vi "csm_lumikki_instron_startRamp_poller.vi"   [LabVIEW 2009]
types:
  T1 = cluster{"Device ID":i32, "Device Name":string, "Device Type":i32}[]
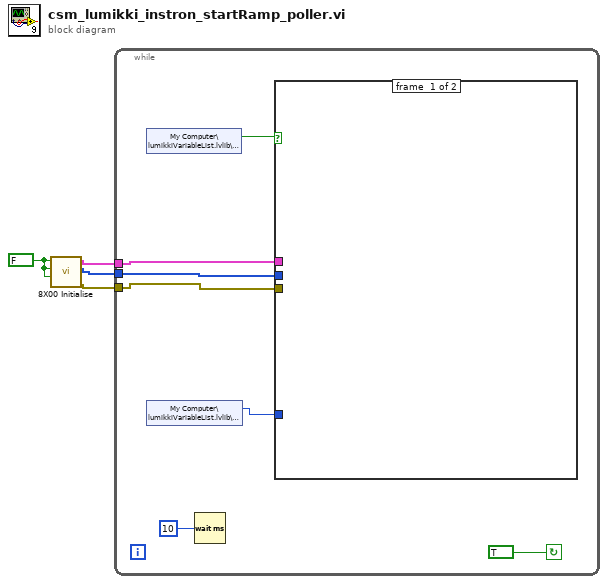
[diagram p0: block diagram]
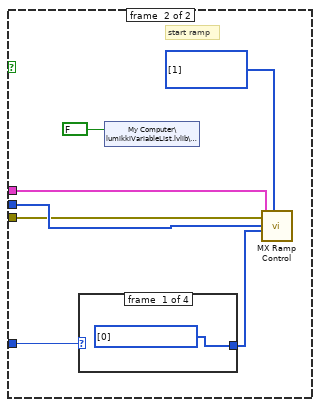
[diagram p2: hidden frame]
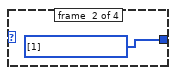
[diagram p3: hidden frame]
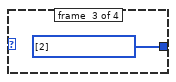
[diagram p4: hidden frame]
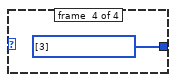
[diagram p5: hidden frame]
diagram:
  w4 = FALSE ("Create Console? (T)")
  n1 = call "8X00 Initialise.vi"("Reset?"=w4, "Create DVM? (T)"=w4, "Create Console? (T)"=w4) -> ("error out"=w1:errorcluster, "Axis Selector"=w2:i32[], "Axis Information"=w3:T1)  [unwired: 1 in, 1 out]
  n2 = while {
    tunnel: w3 -> [w10]
    tunnel: w2 -> [w9]
    tunnel: w1 -> [w8]
    stop <- TRUE continue-if-true
    n3 = shared-variable "My Computer\\lumikkiVariableList.lvlib\\startRamp"() -> (w6:bool)  [unwired: 1 in, 1 out]
    n4 = shared-variable "My Computer\\lumikkiVariableList.lvlib\\channelInt"() -> (w7:i32)  [unwired: 1 in, 1 out]
    n5 = Wait (ms)(milliseconds to wait=u32 10) -> ()  [unwired: 1 out]
    n6 = case shown="True" w6 {
      tunnel: w10 -> [_ w16]
      tunnel: w9 -> [_ w15]
      tunnel: w8 -> [_ w14]
      tunnel: w7 -> [_ w13]
      frame #0 {
      }
      frame #1 {
        w18 = u16[] [1] items=["Stop", "Start or continue", "Hold", "Continue", "Return ramp to set level at fixed rate", "Reserved", "Reserved", "Start Random without demand hold", "Start Random with demand hold", "Prepare Random Start without demand hold", "Prepare Random Start with demand hold", "Unslave", "Reserved", "Reserved", "Start Sample Data Playback or Resume", "Prepare for Start of Sample Data", "Reserved", "Reserved", "Resume Playback", "Start an electromechanical frame return"] ("Ramp Control")
        # "start ramp"
        n7 = case shown="1, Default" w13 {
          tunnel: [w19 w20 w21 w22] -> w17
          frame #0 {
            w19 = u16[] [0] items=["Channel 1", "Channel 2", "Channel 3", "Channel 4"] ("Choose channel to apply\nthe setpoint")
          }
          frame #1 {
            w20 = u16[] [1] items=["Channel 1", "Channel 2", "Channel 3", "Channel 4"] ("Choose channel to apply\nthe setpoint")
          }
          frame #2 {
            w21 = u16[] [2] items=["Channel 1", "Channel 2", "Channel 3", "Channel 4"] ("Choose channel to apply\nthe setpoint")
          }
          frame #3 {
            w22 = u16[] [3] items=["Channel 1", "Channel 2", "Channel 3", "Channel 4"] ("Choose channel to apply\nthe setpoint")
          }
        }
        n8 = shared-variable "My Computer\\lumikkiVariableList.lvlib\\startRamp"(FALSE ("startRamp")) -> ()  [unwired: 1 in, 1 out]
        n9 = call "MX Ramp Control.vi"("Ramp Control"=w18, "error in (no error)"=w14, "Channels In"=w17, "Axis Selector In"=w15, "Axis Information In"=w16) -> ()  [unwired: 2 in, 4 out]
      }
    }
  }
